vi "AO_settings_to_string.vi"(8 "error in":errorcluster, 11 "Analog Output Parameters":T1={"Enable Analog Out?"=TRUE, "Physical Channel"="PXI1Slot2/ao0:3", "Minimum Value"=-10.0, "Maximum Value"=10.0, "Samples per second"=10000.0, "Total AO Time (seconds)"="2.5", "Analog Output Equations for each Channel"=["2+2*spike((t-0.02)/(x/1000))-2*spike((t-0.02-x/1000)/(300/1000))", "-0.4+3.8*spike((t-0.02)/(x/1000))+.75*spike((t-0.02-x/1000)/(300/1000))", "-.35-2.25*spike((t-0.02)/(x/1000))+.6*spike((t-0.02-x/1000)/(300/1000))", "-.95+.35*spike((t-0.02)/(x/1000))-.35*spike((t-0.02-x/1000)/(300/1000))"], "Start Trigger"={"Wait for start trigger?"=TRUE, "source"="/PXI1Slot6/do/StartTrigger", "edge"=10280}} {"Start Trigger"."edge" items=["Rising"=10280, "Falling"=10171]; "Maximum Value" format="%0.2f"; "Minimum Value" format="%0.2f"}) -> (0 "error out":errorcluster, 3 "Analog Output Settings string":string)   [LabVIEW 2012, in "Analog_Output.lvclass"]
uses:
  Analog_Output.lvclass
  AO_settings.ctl
panel:
  # "You may use formulas here.  If 't' is not specified in the variable or parameter tables, it will be used here as time in seconds.\nIn addition to the usual functions (sin(), cos(), etc.) you may also use spike(), square() and step(), \nNote, analog output will continue until Total AO Time runs out, or Measurement Timeout is reached, \neven if HSDIO pulses or DAQmx pulses have finished."
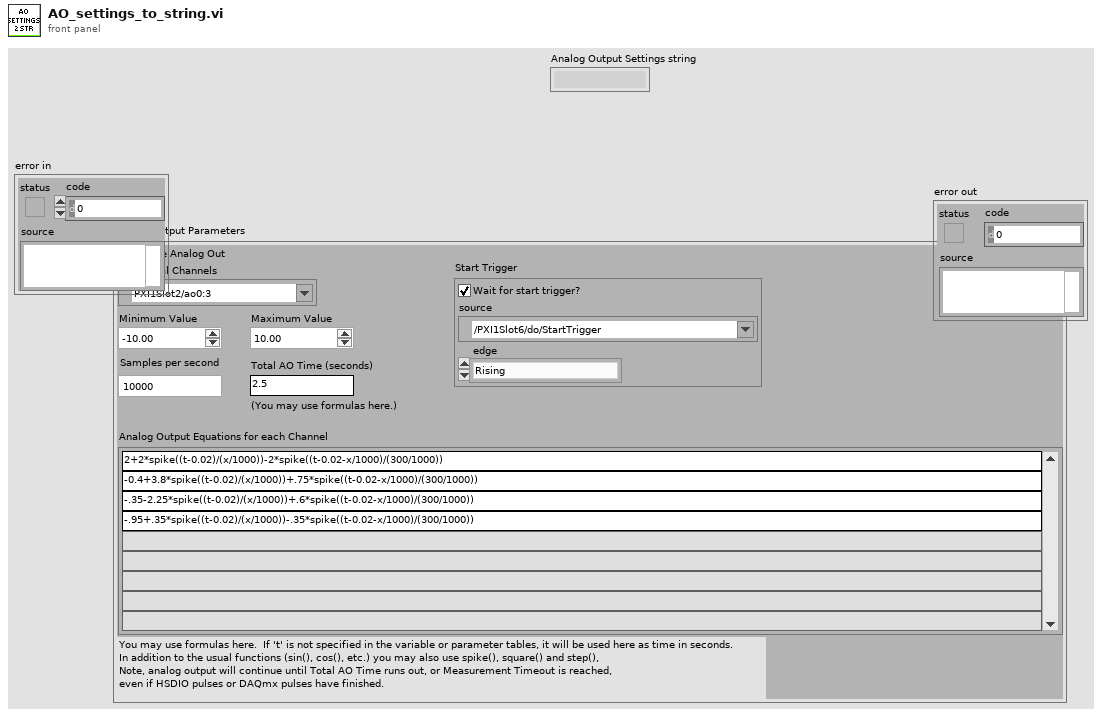
[diagram p1: front panel]
types:
  T1 = typedef "Analog_Output.lvclass/AO_settings.ctl" = cluster{"Enable Analog Out?":bool, "Physical Channel":tag, "Minimum Value":dbl, "Maximum Value":dbl, "Samples per second":dbl, "Total AO Time (seconds)":string, "Analog Output Equations for each Channel":string[], "Start Trigger":cluster{"Wait for start trigger?":bool, "source":tag, "edge":i32}}
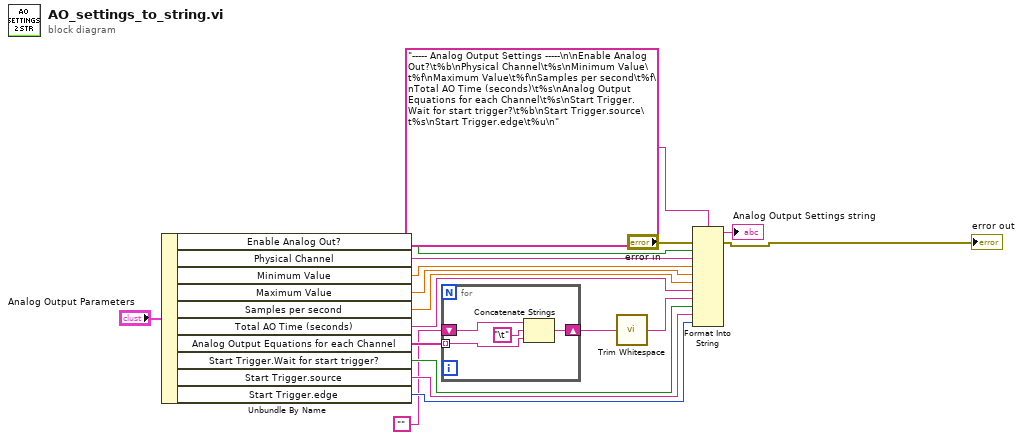
[diagram p0: block diagram]
diagram:
  n1 = Unbundle By Name("Analog Output Parameters") -> ("Enable Analog Out?"=w16:bool, "Physical Channel"=w15:tag, "Minimum Value"=w14:dbl, "Maximum Value"=w13:dbl, "Samples per second"=w12:dbl, "Total AO Time (seconds)"=w11:string, "Analog Output Equations for each Channel"=w7:string[], "Start Trigger.Wait for start trigger?"=w10:bool, "Start Trigger.source"=w9:tag, "Start Trigger.edge"=w8:i32)
  n2 = for {
    tunnel: w7 -> [w20] mode=indexing
    shift-right: [w19] -> w5
    shift-left: "" -> [w22]
    n3 = Concatenate Strings(w22, "\t", w20) -> (w19:string)
  }
  n4 = call <vilib>:"Trim Whitespace.vi"("string"=w5) -> ("trimmed string"=w4:string)  [unwired: 1 in]
  n5 = Format Into String(format string="----- Analog Output Settings -----\n\nEnable Analog Out?\t%b\nPhysical Channel\t%s\nMinimum Value\t%f\nMaximum Value\t%f\nSamples per second\t%f\nTotal AO Time (seconds)\t%s\nAnalog Output Equations for each Channel\t%s\nStart Trigger.Wait for start trigger?\t%b\nStart Trigger.source\t%s\nStart Trigger.edge\t%u\n", error in="error in", w16, w15, w14, w13, w12, w11, w4, w10, w9, w8) -> (resulting string=→"Analog Output Settings string":string, error out=→"error out":errorcluster)  [unwired: 1 in]
